vi "Background Fit and Subtraction.vi"(0 "X":dbl[](array[numeric]), 1 "Y":dbl[](array[numeric])) -> (2 "best fit params":dbl[](array[numeric]), 3 "signal":dbl[](array[numeric]), 4 "background":dbl[](array[numeric]))   [LabVIEW 2015]
doc: "Given a set of x- and y-values and a user-defined form of the background, does a best fit to the background. Returns fitted background as well as signal (i.e., data with background subtracted)."
uses:
  <vilib>/gmath/NumericalOptimization/Nonlinear Curve Fit LM formula string.vi
  <vilib>/gmath/NI_Gmath.lvlib
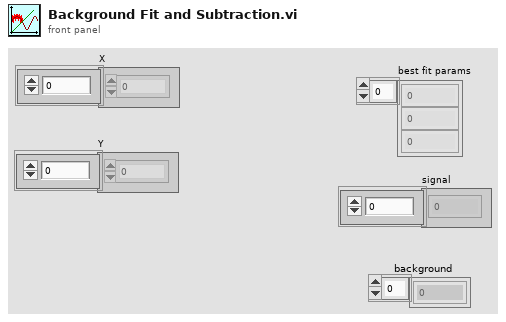
[diagram p1: front panel]
types:
  T1 = cluster{"model":string, "Parameters":string[], "x":string}
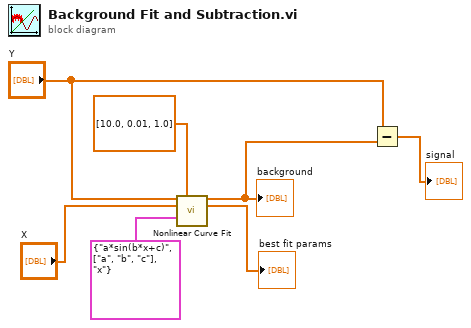
[diagram p0: block diagram]
diagram:
  n1 = call-poly <vilib>:"Nonlinear Curve Fit.vi"("Y"="Y", "initial parameters"=dbl[] [10.0, 0.01, 1.0], "X"="X", "model description"=T1 {"model"="a*sin(b*x+c)", "Parameters"=["a", "b", "c"], "x"="x"}) -> ("best nonlinear fit"=w3:dbl[], "best fit parameters"=→"best fit params":dbl[])  [unwired: 7 in, 3 out]
  "background" <- w3
  n2 = Subtract(x="Y", y=w3) -> (x-y=→"signal":dbl[])
